vi "3onmi.vi"(9 "gear ratio":dbl, 11 "wheel radius":dbl) -> (1 "ccw motor velocity setpoints":dbl[](array[numeric]))   [LabVIEW 2018]
uses:
  <vilib>/robotics/Steering/Wheel/Wheel Parameters.ctl
  <vilib>/robotics/Steering/Wheel/Rotation Direction.ctl
  <vilib>/robotics/Steering/Omnidirectional Wheel/NI_Robotics_Omnidirectional Wheel.lvclass
  C:/Program Files (x86)/National Instruments/LabVIEW 2018/vi.lib/robotics/Steering/Wheel/NI_Robotics_Wheel.lvclass
  <vilib>/robotics/Steering/Omnidirectional Wheel/Create Omnidirectional Wheel.vi
  <vilib>/robotics/Steering/Steering Frame/Create User Defined Steering Frame.vi
  <vilib>/robotics/Steering/Steering Frame/Apply Steering Frame Velocity to Motors.vi
  <vilib>/robotics/Steering/Steering Frame/NI_Robotics_Steering Frame.lvclass
  <vilib>/robotics/Steering/Wheel/NI_Robotics_Wheel.lvclass
panel:
  out "complete":bool
  in  "X Velocity (m/s)":dbl(slide) min=-1.0 max=1.0 scale=-1.0..1.0
  in  "Y Velocity (m/s)":dbl(slide) min=-1.0 max=1.0 scale=-1.0..1.0
  in  "Angular Velocity (rad/s)":dbl(slide) min=-1.0 max=1.0 scale=1.0..-1.0
  out "X Velocity Feedback":dbl(slide) scale=-1.0..1.0
  out "Y Velocity Feedback":dbl(slide) scale=-1.0..1.0
  out "Angular Velocity Feedback":dbl(slide) scale=1.0..-1.0
  in  "stop":bool
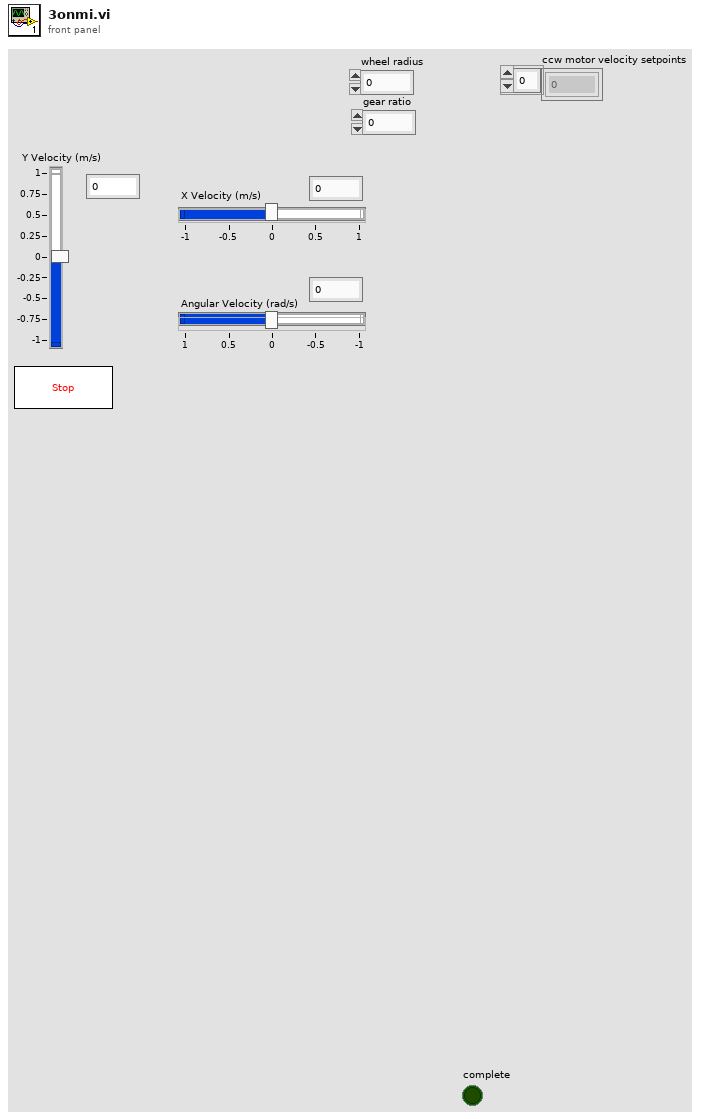
[diagram p1: front panel]
types:
  T1 = typedef "NI_Robotics_Wheel.lvclass/Rotation Direction.ctl" = u16
  T2 = typedef "NI_Robotics_Wheel.lvclass/Wheel Parameters.ctl" = cluster{"wheel radius":dbl, "gear ratio":dbl, "forward rotation direction":T1}
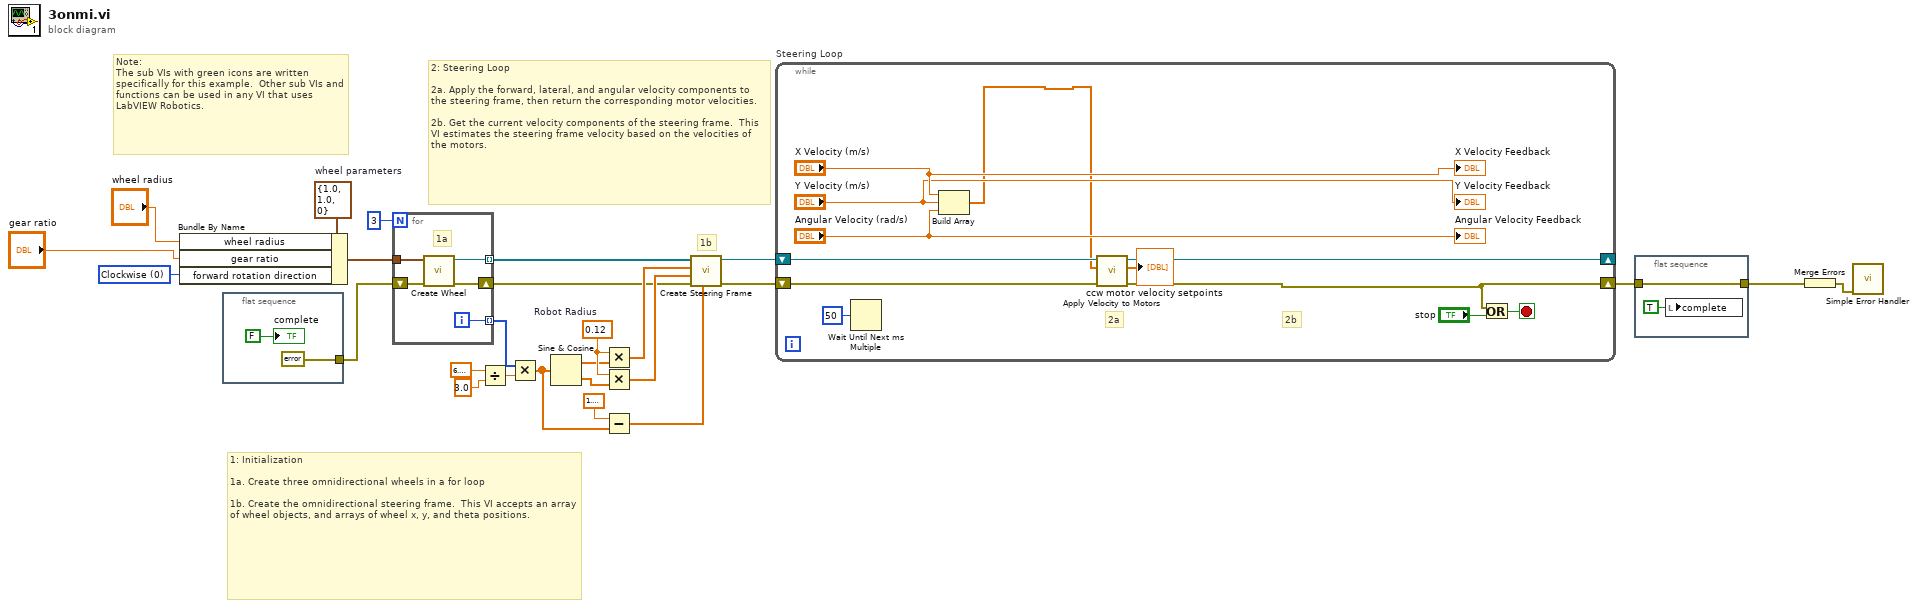
[diagram p0: block diagram]
diagram:
  w9 = T1 0 items=["Clockwise", "Counterclockwise"] ("forward rotation direction")
  w14 = 0.12  # Robot Radius
  w25 = T2 {"wheel radius"=1.0, "gear ratio"=1.0, "forward rotation direction"=0}  # wheel parameters
  # "Note:\nThe sub VIs with green icons are written specifically for this example.  Other sub VIs and functions can be used in any VI that uses LabVIEW Robotics."
  # "2: Steering Loop\n\n2a. Apply the forward, lateral, and angular velocity components to the steering frame, then return the corresponding motor velocities.\n\n2b. Get the current velocity components of the steering frame.  This VI estimates the steering frame velocity based on the velocities of the motors."
  # "1b"
  # "1: Initialization\n\n1a. Create three omnidirectional wheels in a for loop\n\n1b. Create the omnidirectional steering frame.  This VI accepts an array of wheel objects, and arrays of wheel x, y, and theta positions."
  n1 = Bundle By Name(cluster=w25, "wheel radius"="wheel radius", "gear ratio"="gear ratio", "forward rotation direction"=w9) -> (w24:T2)
  n2 = flat-sequence {
    tunnel: [errorcluster {"status"=FALSE, "code"=0, "source"=""} ("error out")] -> w22
    frame #0 {
      "complete" <- FALSE ("complete")
    }
  }
  n3 = for {
    N: 3 -> [_]
    shift-right: [w32] -> w7
    shift-left: w22 -> [w33]
    tunnel: [w31] -> w19 mode=indexing
    tunnel: w24 -> [w30]
    tunnel: [w29] -> w15 mode=indexing
    i -> [w29]
    # "1a"
    n4 = call-poly <vilib>:"Create Wheel.vi"("error in (no error)"=w33, "wheel parameters"=w30) -> ("error out"=w32:errorcluster, "omni wheel out"=w31:refnum<class "NI_Robotics_Omnidirectional Wheel.lvclass">)  [unwired: 8 in]
  }
  n5 = Divide(x=6.283185307179586, y=3.0) -> (x/y=w16:dbl)
  n6 = Multiply(x=w15, y=w16) -> (x*y=w5:dbl[])
  n7 = Sine & Cosine(0:w5) -> (1:w4:dbl[], 2:w3:dbl[])
  n8 = Multiply(x=w14, y=w4) -> (x*y=w13:dbl[])
  n9 = Multiply(x=w14, y=w3) -> (x*y=w12:dbl[])
  n10 = Subtract(x=1.5707963267948966, y=w5) -> (x-y=w10:dbl[])
  n11 = call-poly <vilib>:"Create Steering Frame.vi"("wheel frame angles (rad)"=w10, "error in (no error)"=w7, "wheel y positions"=w12, "wheel x positions"=w13, "wheels"=w19) -> ("error out"=w6:errorcluster, "steering frame out"=w26:refnum<class "NI_Robotics_Steering Frame.lvclass">)  [unwired: 5 in]
  n12 = while "Steering Loop" {
    shift-right: [w40] -> _
    shift-left: w26 -> [w42]
    shift-right: [w39] -> w23
    shift-left: w6 -> [w41]
    stop <- w43 stop-if-true
    # "2b"
    # "2a"
    n13 = Wait Until Next ms Multiple(millisecond multiple=u32 50) -> ()  [unwired: 1 out]
    n14 = Build Array("X Velocity (m/s)", "Y Velocity (m/s)", "Angular Velocity (rad/s)") -> (w35:dbl[])
    n15 = call-poly <vilib>:"Apply Velocity to Motors.vi"("error in (no error)"=w41, "steering frame velocity"=w35, "steering frame in"=w42) -> ("error out"=w39:errorcluster, "ccw motor velocity setpoints"=→"ccw motor velocity setpoints":dbl[], "steering frame out"=w40:refnum<class "NI_Robotics_Steering Frame.lvclass">)  [unwired: 4 in, 2 out]
    n16 = Or(x=w39, y="stop") -> (x .or. y?=w43:bool)
    "X Velocity Feedback" <- "X Velocity (m/s)"
    "Y Velocity Feedback" <- "Y Velocity (m/s)"
    "Angular Velocity Feedback" <- "Angular Velocity (rad/s)"
  }
  n17 = flat-sequence {
    tunnel: w23 -> [w46]
    tunnel: [w46] -> w21
    frame #0 {
      n18 = local write "complete"(TRUE ("complete")) -> ()
    }
  }
  n19 = Merge Errors(w21) -> (w20:errorcluster)
  n20 = call <vilib>:"Simple Error Handler.vi"("error in (no error)"=w20) -> ()  [unwired: 4 in, 5 out]
